vi "Create Error Message.vi"(2 "error in (no error)":errorcluster) -> (4 "Error Message":T1)   [LabVIEW 2021, in "CIFPluginManager.lvclass"]
uses:
  CIFPluginManager.lvclass
  CIFPluginManager.lvclass/CIFPluginManager.ctl
  CIF_Manager_client/RPC Messages/cif_common_Status.ctl
  CIF_Manager_client/CIF_Manager_client.lvlib
  <vilib>/CIF Foundation/CIF Utilities/Errors/Errors_CIF_U.lvlib
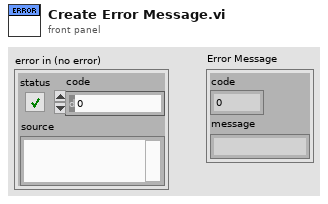
[diagram p1: front panel]
types:
  T1 = typedef "CIF_Manager_client.lvlib/cif_common_Status.ctl" = cluster{"code":i32, "message":string}
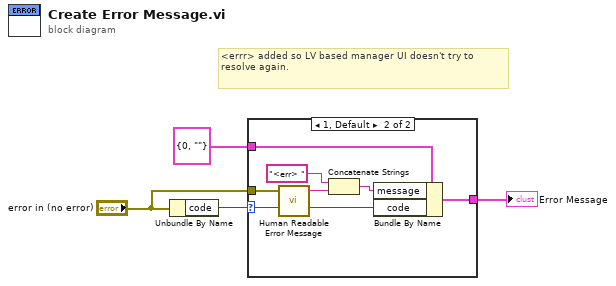
[diagram p0: block diagram]
diagram:
  # "<errr> added so LV based manager UI doesn't try to resolve again."
  n1 = Unbundle By Name("error in (no error)") -> ("code"=w4:i32)
  n2 = case shown="1, Default" w4 {
    selector: w4 -> [_ w10]
    tunnel: "error in (no error)" -> [_ w7]
    tunnel: T1 {"code"=0, "message"=""} ("Error Message 2") -> [w5 w12]
    tunnel: [w5 w11] -> w1
    frame 0 {
    }
    frame 1, Default {
      n3 = call <vilib>:"Human Readable Error Message.vi"("error in (no error)"=w7) -> ("Human readable error message"=w6:string)  [unwired: 4 in]
      n4 = Concatenate Strings("<err> " ("string"), w6) -> (w9:string)
      n5 = Bundle By Name(cluster=w12, "message"=w9, "code"=w10) -> (w11:T1)
    }
  }
  "Error Message" <- w1
